vi "Get SMO HELP getAll.vi"(8 "error in (no error)":errorcluster, 11 "Instrument.Framework-Template in":refnum<class "Instrument.Framework-Template.lvclass">) -> (0 "error out":errorcluster, 1 "response info table":string[][](array[string])=[["name", "description"], ["*", "*"]], 2 "response cluster":variant, 3 "Instrument.Framework-Template out":refnum<class "Instrument.Framework-Template.lvclass">)   [LabVIEW 2019, in "Instrument.Framework-Template.lvclass"]
uses:
  Instrument.Framework-Template.lvclass
  Typedefs/Instrument.Framework-Template.getAll--Cluster.ctl
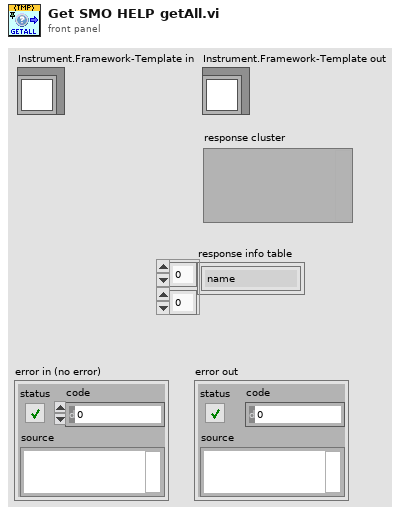
[diagram p1: front panel]
types:
  T1 = typedef "Instrument.Framework-Template.lvclass/Instrument.Framework-Template.getAll--Cluster.ctl" = cluster{"Levy 1":dbl, "Logger SMO":dbl, "SMO Boolean":bool, "SMO String":string}
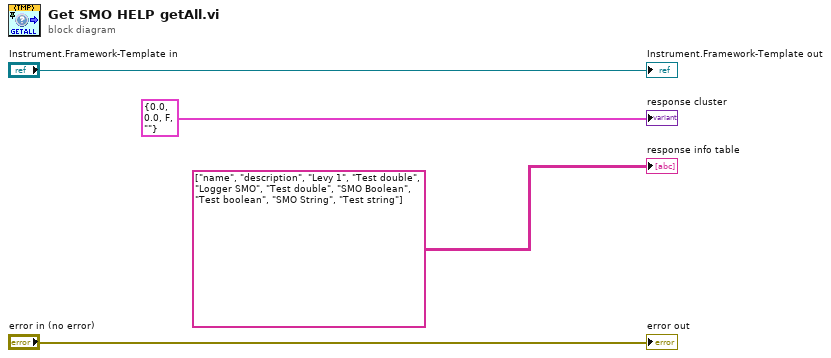
[diagram p0: block diagram]
diagram:
  "Instrument.Framework-Template out" <- "Instrument.Framework-Template in"
  "response info table" <- string[][] [["name", "description"], ["Levy 1", "Test double"], ["Logger SMO", "Test double"], ["SMO Boolean", "Test boolean"], ["SMO String", "Test string"]] ("response/request info table: description of request or reponse cluster")
  "error out" <- "error in (no error)"
  "response cluster" <- T1 {"Levy 1"=0.0, "Logger SMO"=0.0, "SMO Boolean"=FALSE, "SMO String"=""}
